vi "SPCFileNameCheck.vi"() -> ()   [LabVIEW 2012]
uses:
  <vilib>/Utility/SMTP/NI_SMTPEmail.lvlib
panel:
  out "substring 2":string
  out "String 2":string
  out "substring":string
  out "length":i32
  out "String":string
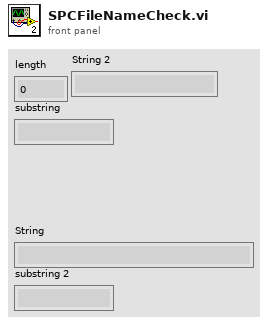
[diagram p1: front panel]
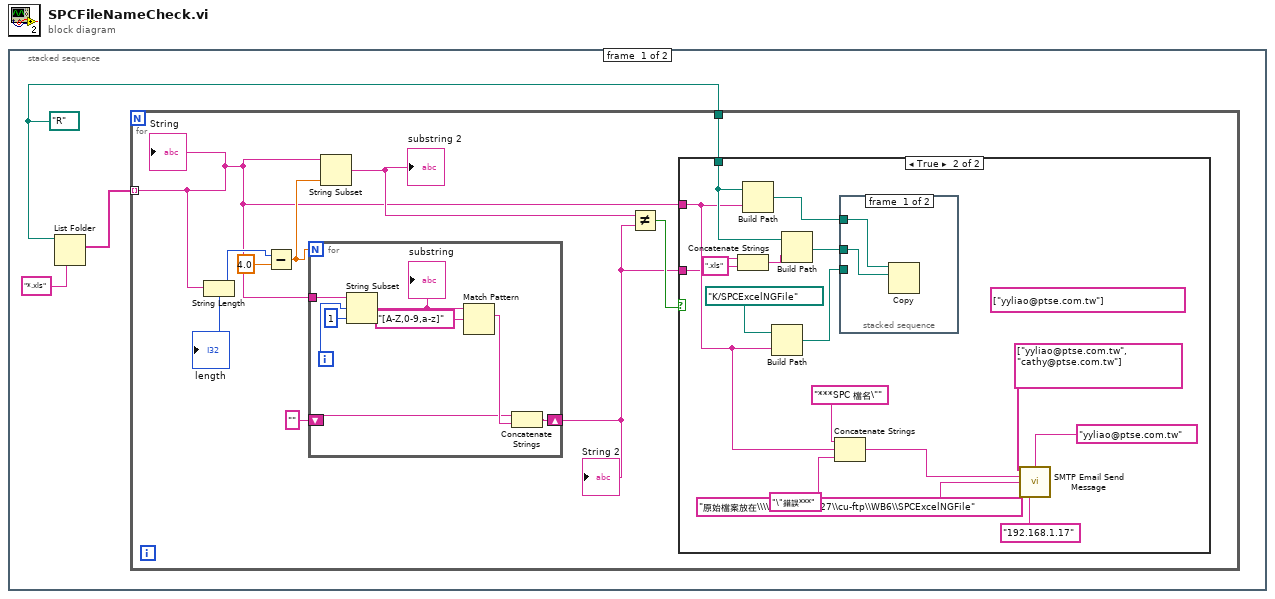
[diagram p0: block diagram]
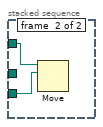
[diagram p3: hidden frame]
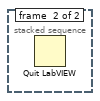
[diagram p4: hidden frame]
diagram:
  n1 = stacked-sequence {
    frame #0 {
      w1 = path "R:/" ("base path")
      n2 = List Folder(path=w1, pattern="*.xls" ("name or relative path")) -> (filenames=w2:string[])  [unwired: 2 in, 3 out]
      n3 = for {
        tunnel: w2 -> [w5] mode=indexing
        tunnel: w1 -> [w6]
        n4 = String Length(string=w5) -> (length=w11:i32)
        "length" <- w11
        n5 = Subtract(x=w11, y=4.0) -> (x-y=w9:dbl)
        n6 = for {
          N: w9 -> [_]
          tunnel: w5 -> [w40]
          shift-right: [w35] -> w4
          shift-left: "" -> [w33]
          i -> [w38]
          n7 = String Subset(string=w40, offset (0)=w38, length (rest)=1 ("length (rest)")) -> (substring=w37:string)
          "substring" <- w37
          n8 = Match Pattern(string=w37, regular expression="[A-Z,0-9,a-z]") -> (match substring=w34:string)  [unwired: 1 in, 3 out]
          n9 = Concatenate Strings(w33, w34) -> (w35:string)
        }
        "String 2" <- w4
        n10 = String Subset(string=w5, length (rest)=w9) -> (substring=w8:string)  [unwired: 1 in]
        "substring 2" <- w8
        n11 = Not Equal?(x=w8, y=w4) -> (x != y?=w7:bool)
        n12 = case shown="True" w7 {
          tunnel: w6 -> [_ w26]
          tunnel: w5 -> [_ w20]
          tunnel: w4 -> [_ w17]
          frame False {
          }
          frame True {
            (unwired) string[] ["yyliao@ptse.com.tw"] ("recipients")
            n13 = Concatenate Strings(w17, ".xls" ("string")) -> (w15:string)
            n14 = Build Path(base path=w26, name or relative path=w20) -> (appended path=w28:path)
            n15 = Build Path(base path=path "K:/SPCExcelNGFile", name or relative path=w20) -> (appended path=w24:path)
            n16 = Build Path(base path=w26, name or relative path=w15) -> (appended path=w25:path)
            n17 = Concatenate Strings("***SPC 檔名\"" ("subject ([No Subject])"), w20, "\"錯誤***" ("string")) -> (w19:string)
            n18 = stacked-sequence {
              tunnel: w28 -> [w30 w32]
              tunnel: w25 -> [w29 _]
              tunnel: w24 -> [_ w31]
              frame #0 {
                n19 = Copy(10:w29, 11:w30) -> ()  [unwired: 3 in, 3 out]
              }
              frame #1 {
                n20 = Move(source path=w32, 10:w31) -> ()  [unwired: 3 in, 3 out]
              }
            }
            n21 = call <vilib>:"SMTP Email Send Message.vi"("recipients"=string[] ["yyliao@ptse.com.tw", "cathy@ptse.com.tw"], "mail server"="192.168.1.17", "return address"="yyliao@ptse.com.tw", "subject ([No Subject])"=w19, "message"="原始檔案放在\\\\192.168.1.27\\cu-ftp\\WB6\\SPCExcelNGFile") -> ()  [unwired: 9 in, 2 out]
          }
        }
        "String" <- w5
      }
    }
    frame #1 {
      n22 = Quit LabVIEW() -> ()  [unwired: 1 in]
    }
  }
